vi "Autonomous Independent.vi"   [LabVIEW 2013]
doc: "This VI is called when autonomous begins, and will automatically be terminated when autonomous ends. You can carry out timed or sensor driven robot movement independently without needing to return to the caller."
uses:
  Robot Global Data.vi
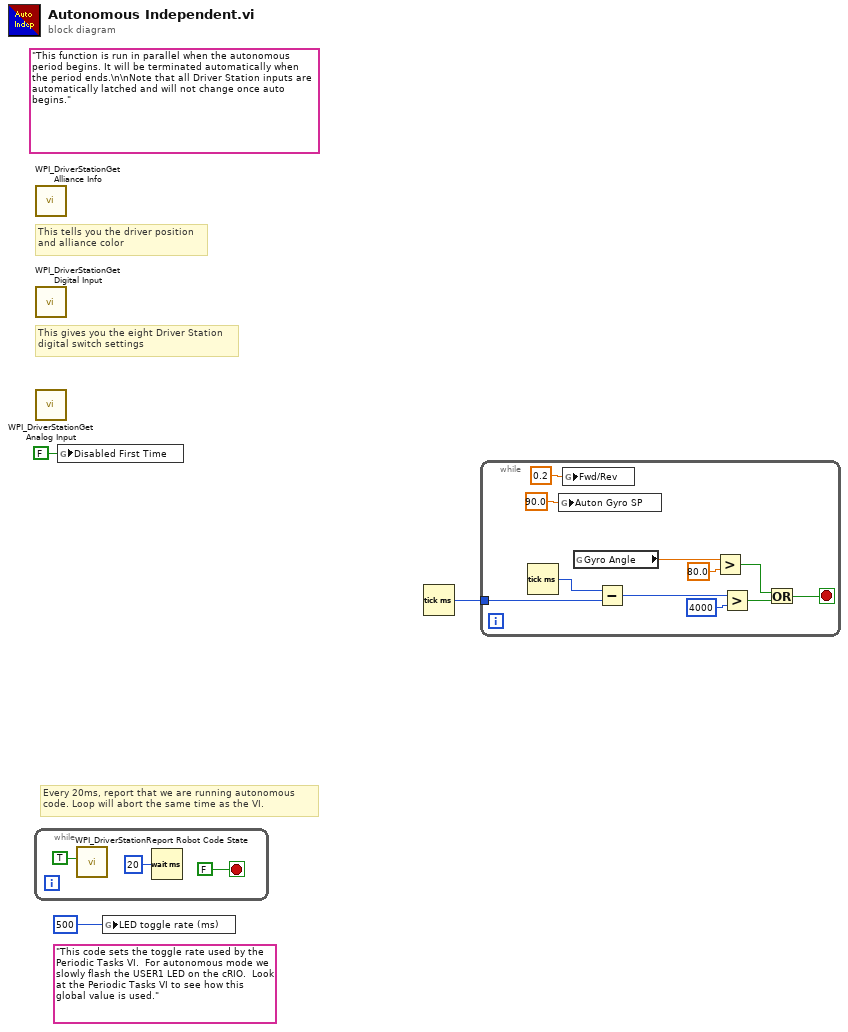
[diagram p0: block diagram]
diagram:
  (unwired) "This code sets the toggle rate used by the Periodic Tasks VI.  For autonomous mode we slowly flash the USER1 LED on the cRIO.  Look at the Periodic Tasks VI to see how this global value is used."
  (unwired) "This function is run in parallel when the autonomous period begins. It will be terminated automatically when the period ends.\n\nNote that all Driver Station inputs are automatically latched and will not change once auto begins."
  # "Every 20ms, report that we are running autonomous\ncode. Loop will abort the same time as the VI."
  # "This tells you the driver position\nand alliance color"
  # "This gives you the eight Driver Station\ndigital switch settings"
  n1 = while {
    stop <- FALSE stop-if-true
    n2 = call <vilib>:"WPI_DriverStationReport Robot Code State.vi"("Autonomous"=TRUE) -> ()  [unwired: 10 in, 1 out]
    n3 = Wait (ms)(milliseconds to wait=u32 20) -> ()  [unwired: 1 out]
  }
  n4 = call <vilib>:"WPI_DriverStationGet Alliance Info.vi"() -> ()  [unwired: 12 out]
  n5 = call <vilib>:"WPI_DriverStationGet Digital Input.vi"() -> ()  [unwired: 12 out]
  n6 = call <vilib>:"WPI_DriverStationGet Analog Input.vi"() -> ()  [unwired: 12 out]
  n7 = global write "Robot Global Data.vi" "Disabled First Time"(FALSE ("Disabled First Time")) -> ()
  n8 = global write "Robot Global Data.vi" "LED toggle rate (ms)"(u32 500 ("LED ms toggle rate")) -> ()
  n9 = Tick Count (ms)() -> (millisecond timer value=w1:u32)
  n10 = while {
    tunnel: w1 -> [w8]
    stop <- w7 stop-if-true
    n11 = Tick Count (ms)() -> (millisecond timer value=w12:u32)
    n12 = global write "Robot Global Data.vi" "Auton Gyro SP"(90.0 ("Auton Gyro SP")) -> ()
    n13 = global write "Robot Global Data.vi" "Fwd/Rev"(0.2 ("Fwd/Rev")) -> ()
    n14 = global read "Robot Global Data.vi" "Gyro Angle"() -> (w16:dbl)
    n15 = Subtract(x=w12, y=w8) -> (x-y=w11:u32)
    n16 = Greater?(x=w16, y=80.0) -> (0:w14:bool)
    n17 = Greater?(x=w11, y=u32 4000) -> (0:w10:bool)
    n18 = Or(x=w14, y=w10) -> (x .or. y?=w7:bool)
  }
